vi "Set Wheel Radius.vi"(6 "subpanel to main command event":T1, 8 "error in (no error)":errorcluster, 10 "wheel radius":dbl, 11 "steering frame ref in":refnum<data-value>) -> (0 "error out":errorcluster, 3 "steering frame ref out":refnum<data-value>)   [LabVIEW 2017, in "NI_Robotics_Configure Steering Frame.lvlib" / "Differential Frame Subpanel.lvlib"]
uses:
  <vilib>/robotics/Dialog/Configure Steering Frame/Differential Frame Subpanel/Differential Frame Subpanel.lvlib
  <vilib>/robotics/Steering/Differential Steering Frame/NI_Robotics_Differential Steering Frame.lvclass
  c:/Program Files (x86)/National Instruments/LabVIEW 2017/vi.lib/robotics/Steering/Steering Frame/NI_Robotics_Steering Frame.lvclass
  <vilib>/robotics/Dialog/Configure Steering Frame/Subpanel to Main Command Event.ctl
  <vilib>/robotics/Dialog/Configure Steering Frame/Subpanel to Main Command.ctl
  <vilib>/robotics/Dialog/Configure Steering Frame/Generate Subpanel to Main Event.vi
  <vilib>/robotics/Steering/Steering Frame/NI_Robotics_Steering Frame.lvclass
  <vilib>/robotics/Dialog/Configure Steering Frame/NI_Robotics_Configure Steering Frame.lvlib
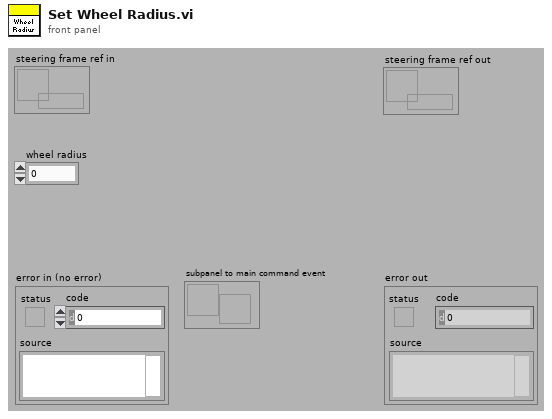
[diagram p1: front panel]
types:
  T1 = typedef "NI_Robotics_Configure Steering Frame.lvlib/Subpanel to Main Command Event.ctl" = refnum<user-event>
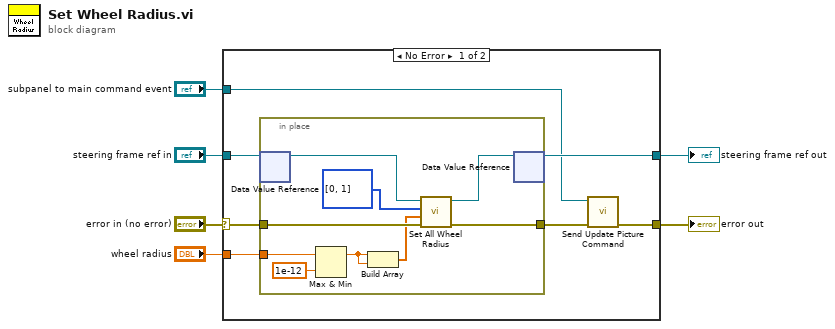
[diagram p0: block diagram]
diagram:
  n1 = case shown="No Error" "error in (no error)" {
    selector: "error in (no error)" -> [w11 w23]
    tunnel: "steering frame ref in" -> [w13 w24]
    tunnel: [w12 w24] -> w4
    tunnel: [w7 w23] -> w3
    tunnel: "wheel radius" -> [w10 _]
    tunnel: "subpanel to main command event" -> [w9 _]
    frame No Error {
      n2 = in-place {
        in-place-border: w11 -> [w20]
        in-place-border: w10 -> [w16]
        in-place-border: [w19] -> w8
        n3 = in-place-dvr #1(w13) -> (w22:refnum<class "NI_Robotics_Differential Steering Frame.lvclass">)  [unwired: 1 out]
        n4 = Max & Min(x=w16, y=1e-12) -> (max(x,y)=w15:dbl)  [unwired: 1 out]
        n5 = Build Array(w15, w15) -> (w17:dbl[])
        n6 = call <vilib>:"Set All Wheel Radius.vi"("error in (no error)"=w20, "wheel radius"=w17, "wheel indexes"=i32[] [0, 1], "steering frame in"=w22) -> ("error out"=w19:errorcluster, "steering frame out"=w21:refnum<class "NI_Robotics_Differential Steering Frame.lvclass">)  [unwired: 5 in, 1 out]
        n7 = in-place-dvr #1(w21) -> (w12:refnum<data-value>)  [unwired: 1 out]
      }
      n8 = call <vilib>:"Send Update Picture Command.vi"("error in (no error)"=w8, "subpanel to main command event"=w9) -> ("error out"=w7:errorcluster)  [unwired: 9 in]
    }
    frame Error {
    }
  }
  "steering frame ref out" <- w4
  "error out" <- w3
